vi "Test.vi"() -> ()   [LabVIEW 2016, in "LS218.lvlib"]
uses:
  LS218.lvlib
  <instrlib>/Lake Shore Cryotronics 218/Lake Shore Cryotronics 218.lvlib
panel:
  in  "VISA resource name":refnum<visa-resource-name>="LS218TS"
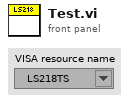
[diagram p1: front panel]
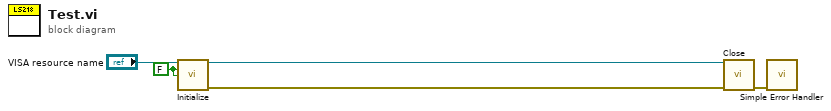
[diagram p0: block diagram]
diagram:
  w3 = FALSE ("ID Query (T: Check)")
  n1 = call <instrlib>:"Initialize.vi"("VISA resource name"="VISA resource name", "ID Query (T: Check)"=w3, "Reset (T: Reset)"=w3) -> ("VISA resource name out"=w2:refnum<visa-resource-name>, "error out"=w1:errorcluster)  [unwired: 11 in]
  n2 = call <instrlib>:"Close.vi"("VISA resource name"=w2, "error in (no error)"=w1) -> ("error out"=w4:errorcluster)  [unwired: 13 in]
  n3 = call <vilib>:"Simple Error Handler.vi"("error in (no error)"=w4) -> ()  [unwired: 4 in, 5 out]
